vi "codegen2.vi"(11 "Arguments":string[](array[string])) -> (2 "Output/Failure Message":string, 3 "Exit Code":i32)   [LabVIEW 2020]
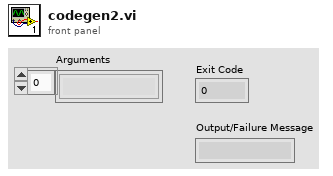
[diagram p1: front panel]
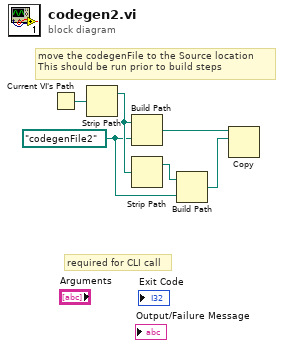
[diagram p0: block diagram]
diagram:
  w3 = path "codegenFile2" ("name or relative path")
  # "required for CLI call"
  # "move the codegenFile to the Source location\nThis should be run prior to build steps"
  n1 = Current VI's Path() -> (path=w6:path)
  n2 = Strip Path(path=w6) -> (stripped path=w5:path)  [unwired: 1 out]
  n3 = Build Path(base path=w5, name or relative path=w3) -> (appended path=w1:path)
  n4 = Strip Path(path=w5) -> (stripped path=w4:path)  [unwired: 1 out]
  n5 = Build Path(base path=w4, name or relative path=w3) -> (appended path=w2:path)
  n6 = Copy(10:w2, 11:w1) -> ()  [unwired: 3 in, 3 out]
